vi "Configure - Analog.vi"(8 "error in (no error)":errorcluster, 10 "digital generation":T1={"data channel list"="", "master clock channel list"="", "digital protocol settings"={"logic level"=enum."3.3 V", "PCM Data Configuration"={"Frame Sync Edge for Channel 0"=enum."Falling", "Channel Count Per Frame"=2, "Channel Length"=32, "Bit Depth"=24, "Channel 0 Offset"=1, "Endianness"=enum."MSB First", "Data Justification"=enum."Left Justified"}, "bit clock rate"=3025000.0, "master clock rate"=3025000.0, "clock mode"=enum."divided clock", "Frame Sync Clock Control"={"Frame Length"=64, "Frame Sync Pulse Width"=32, "Bit Clock Edge  Sync"=enum."Falling"}}, "signal parameters"={"cyclic signal"=[], "channel parameters"=[]}} {"digital protocol settings"."master clock rate" format="%.4p"; "digital protocol settings"."bit clock rate" format="%.4p"}, 11 "AudioGeneration in":refnum<class "AudioGeneration.lvclass">) -> (0 "error out":errorcluster, 3 "AudioGeneration out":refnum<class "AudioGeneration.lvclass">)   [LabVIEW 2021, in "AudioGeneration.lvclass"]
uses:
  AudioGeneration.lvclass
  controls/digital generation settings.ctl
  controls/digital protocol settings.ctl
  <vilib>/PDM Acquisition Toolkit/host/Classes/Session/Controls/Logic Levels.ctl
  <vilib>/PDM Acquisition Toolkit/shared/controls/PCM Data Format Configuration.ctl
  <vilib>/PDM Acquisition Toolkit/shared/controls/Digital Edge.ctl
  <vilib>/PDM Acquisition Toolkit/shared/controls/PCM Bit Endianness.ctl
  <vilib>/PDM Acquisition Toolkit/shared/controls/PCM Data Justification.ctl
  <vilib>/PDM Acquisition Toolkit/shared/controls/clock mode.ctl
  <vilib>/PDM Acquisition Toolkit/shared/controls/PCM Frame Sync Control.ctl
  <vilib>/PDM Acquisition Toolkit/host/Classes/Tasks/I2S Output/Control/SignalProperties.ctl
  <vilib>/PDM Acquisition Toolkit/host/Classes/Channels/I2S Ouput/Controls/GenerationChannelProperties.ctl
  <vilib>/NI/STM/TCP/TCP Write Options.ctl
  controls/generation type.ctl
  <vilib>/NI/STM/TCP/Write Message (TCP).vi
  AudioGeneration.lvclass/AudioGeneration.ctl
  <vilib>/NI/STM/NI STM.lvlib
  controls/AudioGenTypeDefs.lvlib
  <vilib>/PDM Acquisition Toolkit/host/Classes/Session/DecoderSession.lvclass
  <vilib>/PDM Acquisition Toolkit/shared/PDM Shared.lvlib
  <vilib>/PDM Acquisition Toolkit/host/Classes/Channels/I2S Ouput/I2S Output Channel.lvclass
  <vilib>/PDM Acquisition Toolkit/host/Classes/Tasks/I2S Output/I2S Output Task.lvclass
panel:
  out "timeout":bool
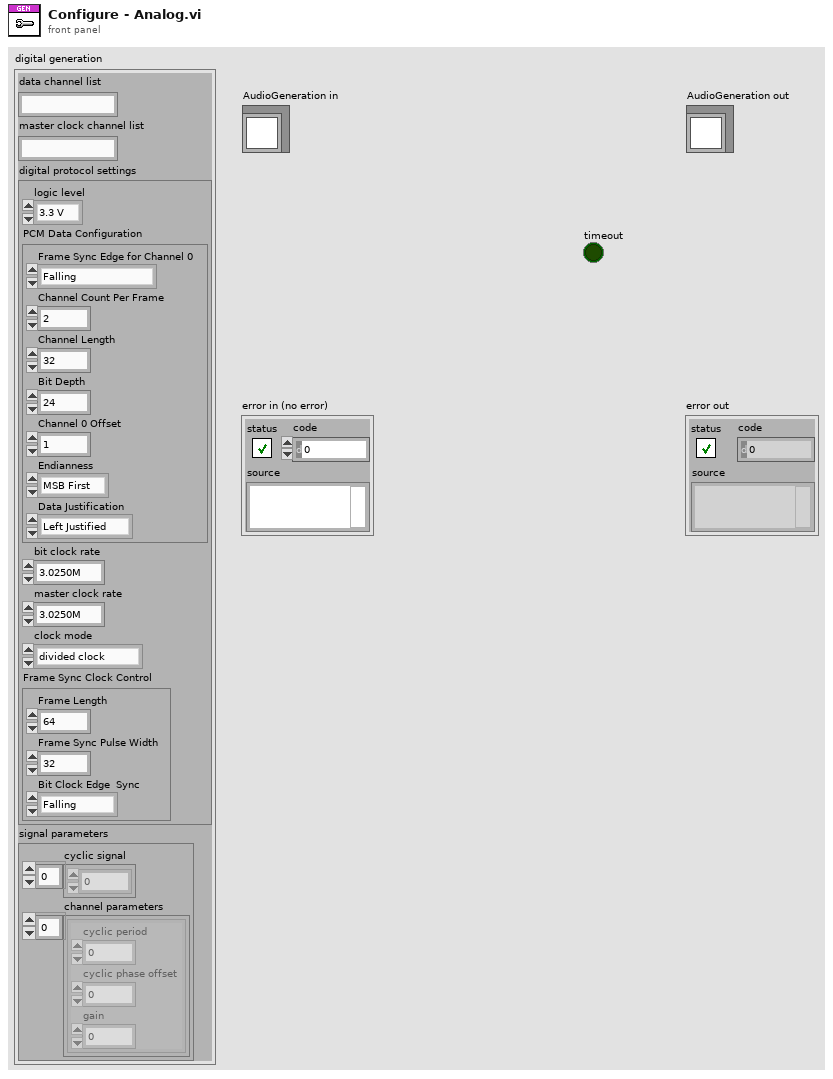
[diagram p1: front panel]
types:
  T1 = typedef "AudioGenTypeDefs.lvlib/digital generation settings.ctl" = cluster{"data channel list":string, "master clock channel list":string, "digital protocol settings":T2, "signal parameters":T10}
  T2 = typedef "AudioGenTypeDefs.lvlib/digital protocol settings.ctl" = cluster{"logic level":T3, "PCM Data Configuration":T4, "bit clock rate":sgl, "master clock rate":sgl, "clock mode":T8, "Frame Sync Clock Control":T9}
  T3 = typedef "PDM Acquisition Class Library.lvlib/DecoderSession.lvclass/Logic Levels.ctl" = enum16{"3.3 V", "1.8 V", "1.2 V"}
  T4 = typedef "PDM Shared.lvlib/PCM Data Format Configuration.ctl" = cluster{"Frame Sync Edge for Channel 0":T5, "Channel Count Per Frame":u8, "Channel Length":u16, "Bit Depth":u8, "Channel 0 Offset":u16, "Endianness":T6, "Data Justification":T7}
  T5 = typedef "PDM Shared.lvlib/Digital Edge.ctl" = enum8{"Rising", "Falling"}
  T6 = typedef "PDM Shared.lvlib/PCM Bit Endianness.ctl" = enum16{"MSB First", "LSB First"}
  T7 = typedef "PDM Shared.lvlib/PCM Data Justification.ctl" = enum16{"Left Justified", "Right Justified"}
  T8 = typedef "PDM Shared.lvlib/clock mode.ctl" = enum16{"divided clock", "DDS"}
  T9 = typedef "PDM Shared.lvlib/PCM Frame Sync Control.ctl" = cluster{"Frame Length":u16, "Frame Sync Pulse Width":u16, "Bit Clock Edge  Sync":T5}
  T10 = typedef "PDM Acquisition Class Library.lvlib/I2S Output Task.lvclass/SignalProperties.ctl" = cluster{"cyclic signal":dbl[], "channel parameters":T11[]}
  T11 = typedef "PDM Acquisition Class Library.lvlib/I2S Output Channel.lvclass/GenerationChannelProperties.ctl" = cluster{"cyclic period":dbl, "cyclic phase offset":dbl, "gain":dbl}
  T12 = typedef "AudioGenTypeDefs.lvlib/generation type.ctl" = enum16{"analog", "digital"}
  T13 = typedef "NI STM.lvlib/TCP Write Options.ctl" = cluster{"ignore timeout error":bool, "timeout ms (1000)":i32}
  T14 = typedef "NI STM.lvlib/TCP Connection Info.ctl" = cluster{"connection ID":refnum<k5>, "meta data":T15[]}
  T15 = typedef "NI STM.lvlib/MetaDataElement.ctl" = string
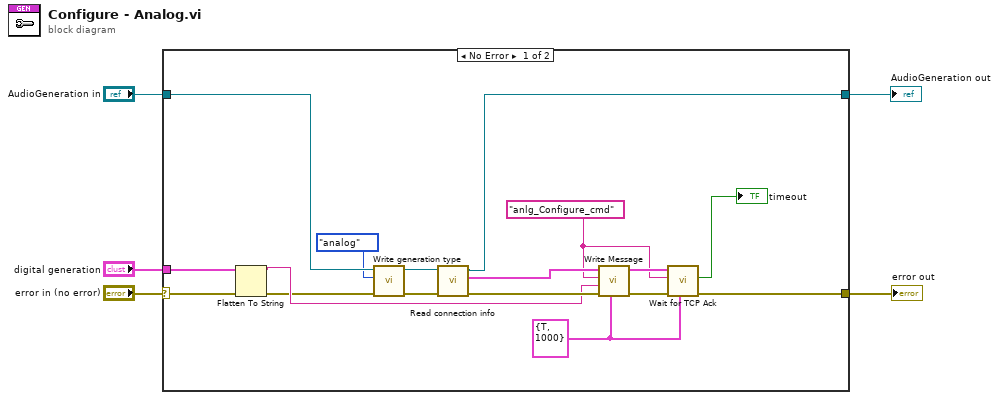
[diagram p0: block diagram]
diagram:
  n1 = case shown="No Error" "error in (no error)" {
    selector: "error in (no error)" -> [w17 w24]
    tunnel: [w19 w24] -> w3
    tunnel: "AudioGeneration in" -> [w11 w23]
    tunnel: [w18 w23] -> w2
    tunnel: "digital generation" -> [w15 _]
    frame No Error {
      w7 = "anlg_Configure_cmd" ("name")
      w8 = T13 {"ignore timeout error"=TRUE, "timeout ms (1000)"=1000} ("options")
      n2 = Flatten To String(anything=w15, error in (no error)=w17) -> (data string=w16:string, error out=w14:errorcluster)  [unwired: 2 in, 1 out]
      n3 = call-dynamic "Write generation type.vi"("error in (no error)"=w14, "generation type"=generation_type."analog", "AudioGeneration in"=w11) -> ("error out"=w13:errorcluster, "AudioGeneration out"=w12:refnum<class "AudioGeneration.lvclass">)  [unwired: 7 in]
      n4 = call-dynamic "Read connection info.vi"("error in (no error)"=w13, "AudioGeneration in"=w12) -> ("error out"=w21:errorcluster, "connection info"=w22:T14, "AudioGeneration out"=w18:refnum<class "AudioGeneration.lvclass">)  [unwired: 7 in]
      n5 = call-poly <vilib>:"Write Message.vi"("options"=w8, "error in"=w21, "data"=w16, "name"=w7, "connection info in"=w22) -> ("error out"=w20:errorcluster, "connection info out"=w9:T14)  [unwired: 5 in]
      n6 = call "Wait for TCP Ack.vi"("options"=w8, "error in (no error)"=w20, "cmd name"=w7, "connection info in"=w9) -> ("error out"=w19:errorcluster, "timeout"=→"timeout":bool)  [unwired: 4 in, 2 out]
    }
    frame Error {
    }
  }
  "error out" <- w3
  "AudioGeneration out" <- w2
